vi "String to Time.vi"(8 "error in (no error)":errorcluster, 11 "String":string) -> (0 "error out":errorcluster, 3 "Time Stamp":timestamp format="%<%X\n%Y/%m/%d>T")   [LabVIEW 2017]
panel:
  # "2020-09-07 22:56:14"
  # "2020-09-08 0:06:51"
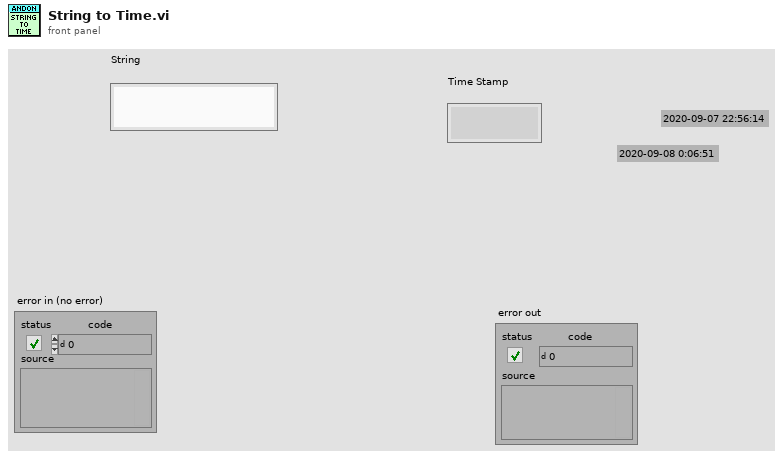
[diagram p1: front panel]
types:
  T1 = cluster{"second":i32, "minute":i32, "hour":i32, "day of month":i32, "month":i32, "year":i32, "day of week":i32, "day of year":i32, "is DST":i32}
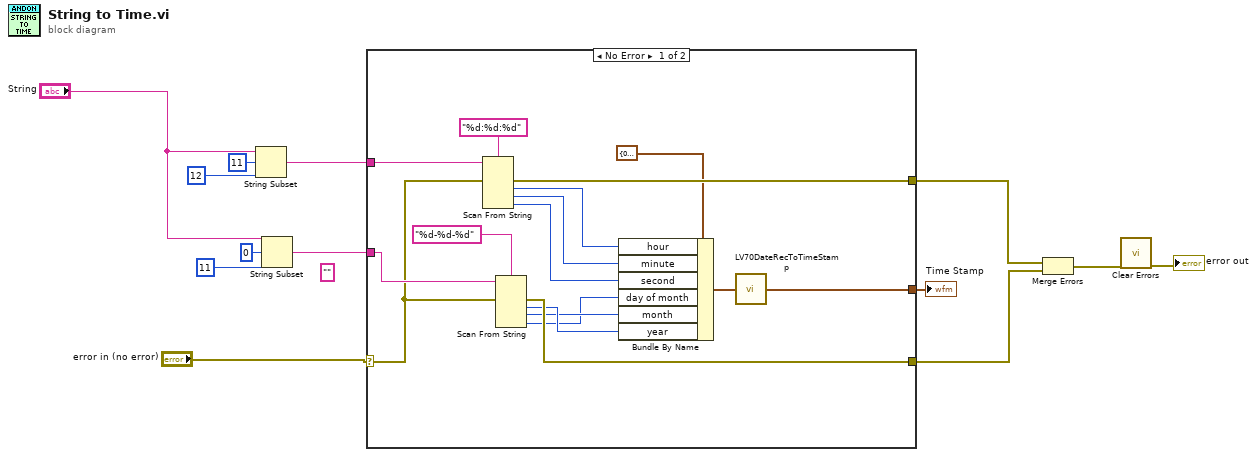
[diagram p0: block diagram]
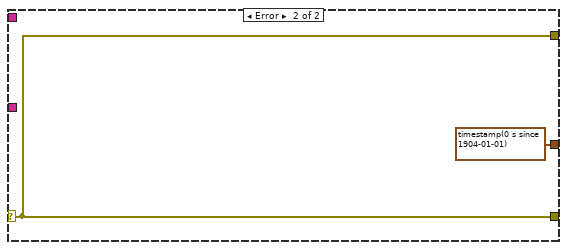
[diagram p2: hidden frame]
diagram:
  (unwired) "" ("substring")
  n1 = String Subset(string="String", offset (0)=11, length (rest)=12 ("length (rest)")) -> (substring=w7:string)
  n2 = String Subset(string="String", offset (0)=0, length (rest)=11 ("length (rest)")) -> (substring=w6:string)
  n3 = case shown="No Error" "error in (no error)" {
    selector: "error in (no error)" -> [w26 w30]
    tunnel: [w18 w30] -> w3
    tunnel: w7 -> [w29 _]
    tunnel: w6 -> [w28 _]
    tunnel: [w25 w30] -> w4
    tunnel: [w19 timestamp(0 s since 1904-01-01) ("Time Stamp")] -> w5
    frame No Error {
      n4 = Scan From String(format string="%d:%d:%d", input string=w29, error in=w26) -> (error out=w25:errorcluster, output 1=w22:i32, output 2=w21:i32, output 3=w20:i32)  [unwired: 4 in, 2 out]
      n5 = Scan From String(format string="%d-%d-%d", input string=w28, error in=w26) -> (error out=w18:errorcluster, output 1=w16:i32, output 2=w15:i32, output 3=w14:i32)  [unwired: 4 in, 2 out]
      n6 = Bundle By Name(cluster=T1 {"second"=0, "minute"=0, "hour"=0, "day of month"=1, "month"=1, "year"=2018, "day of week"=0, "day of year"=0, "is DST"=0} ("date time rec"), "hour"=w22, "minute"=w21, "second"=w20, "day of month"=w14, "month"=w15, "year"=w16) -> (w23:T1)
      n7 = call <vilib>:"LV70DateRecToTimeStamp.vi"("date time rec"=w23) -> ("Time Stamp"=w19:timestamp)
    }
    frame Error {
    }
  }
  "Time Stamp" <- w5
  n8 = Merge Errors(w4, w3) -> (w2:errorcluster)
  n9 = call <vilib>:"Clear Errors.vi"("error in (no error)"=w2) -> ("error out"=→"error out":errorcluster)  [unwired: 5 in, 1 out]
